vi "solar_cfg Write File (Section).vi"(0 "Config Path (*.ini)":path, 1 "Section (\"\" = Use Filename)":string, 2 "Comment":string, 11 "error in (no error)":errorcluster) -> (4 "Config Path out":path, 10 "Found?":bool, 15 "error out":errorcluster)   [LabVIEW 2018]
doc: "Create a configure file section '[SECTION]'. The comment is only written if the section does not exist."
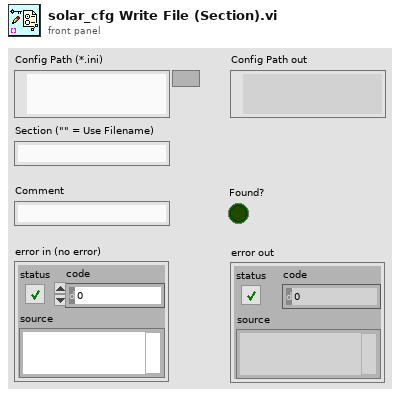
[diagram p1: front panel]
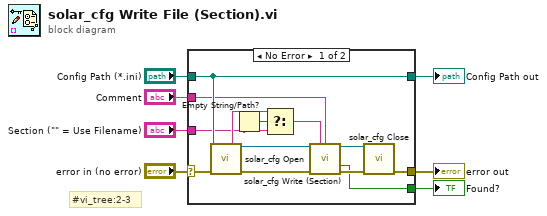
[diagram p0: block diagram]
diagram:
  # "#vi_tree:2-3"
  n1 = case shown="No Error" "error in (no error)" {
    selector: "error in (no error)" -> [w20 w22]
    tunnel: "Config Path (*.ini)" -> [w19 w21]
    tunnel: [w15 w22] -> w5
    tunnel: "Section (\"\" = Use Filename)" -> [w10 _]
    tunnel: [w14 _] -> w3
    tunnel: [w19 w21] -> w2
    tunnel: "Comment" -> [w8 _]
    frame No Error {
      n2 = call "solar_cfg Open.vi"("Config Path (*.ini)"=w19, "error in (no error)"=w20) -> ("Filename"=w12:string, "Config Refnum"=w16:refnum<data-value>, "error out"=w18:errorcluster)  [unwired: 10 in, 1 out]
      n3 = Empty String/Path?(string/path=w10) -> (empty?=w13:bool)
      n4 = Select(t=w12, s=w13, f=w10) -> (s? t:f=w11:string)
      n5 = call "solar_cfg Write (Section).vi"("Config Refnum in"=w16, "Section"=w11, "Comment (New section only)"=w8, "error in (no error)"=w18) -> ("Config Refnum out"=w9:refnum<data-value>, "Found?"=w14:bool, "error out"=w17:errorcluster)  [unwired: 9 in]
      n6 = call "solar_cfg Close.vi"("Config Refnum"=w9, "error in (no error)"=w17) -> ("error out"=w15:errorcluster)  [unwired: 12 in, 1 out]
    }
    frame Error {
    }
  }
  "error out" <- w5
  "Config Path out" <- w2
  "Found?" <- w3
